vi "Teleop.vi"(10 "Match Info":T1={"Autonomous Elapsed Seconds"=0.0, "TeleOp Elapsed Seconds"=0.0, "Disabled Elapsed Seconds"=0.0, "Visited Autonomous"=FALSE, "Visited TeleOp"=FALSE, "Visited Disabled"=FALSE, "Autonomous Settings"={"Autonomous Style"=enum."Independent", "VI Refnum"=refnum}}, 11 "Call Context":T2) -> ()   [LabVIEW 2015]
doc: "This VI is called for each TeleOp packet received from the DS where the robot is not disabled. It is often used to read from the joysticks and update I/O or to update setpoints for timed control loops. It should complete and return within 20 milliseconds or it may miss DS packets."
uses:
  <vilib>/Rock Robotics/WPI/DriverStation/WPI_DriverStationDerivedRobotMode.ctl
  <vilib>/Rock Robotics/WPI/DriverStation/WPI_DriverStationMatch Info.ctl
  <vilib>/Rock Robotics/WPI/Utilities/WPI_GetSetVariantRefNum.vi
  Robot Global Data.vi
  <vilib>/Rock Robotics/Network Tables/NT Write Boolean Array.vi
  <vilib>/Rock Robotics/Network Tables/NT Write Numeric Array.vi
  <vilib>/Rock Robotics/Network Tables/NT Write Boolean.vi
  <vilib>/Rock Robotics/WPI/RobotDrive/WPI_RobotDriveArcadeDrive_Standard(NoSaturation).vi
  <vilib>/Rock Robotics/Network Tables/NT Read Boolean.vi
  <vilib>/Rock Robotics/Network Tables/NT Read Number.vi
panel:
  in  "command limit":dbl=0.25
  out "Sample Slider 0":dbl(slide) scale=0.0..5.0
  out "Sample Boolean 1":bool
  out "Sample Boolean 0":bool
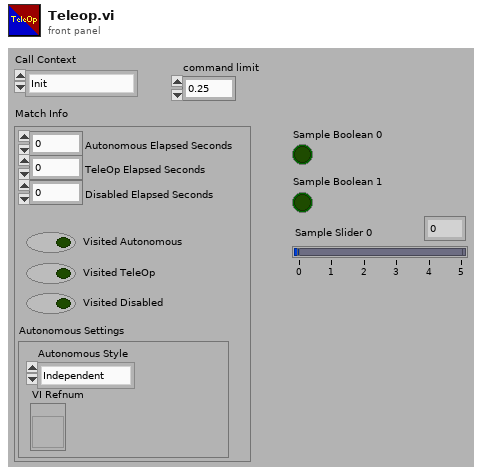
[diagram p1: front panel]
types:
  T1 = typedef "WPI_DriverStationMatch Info.ctl" = cluster{"Autonomous Elapsed Seconds":dbl, "TeleOp Elapsed Seconds":dbl, "Disabled Elapsed Seconds":dbl, "Visited Autonomous":bool, "Visited TeleOp":bool, "Visited Disabled":bool, "Autonomous Settings":cluster{"Autonomous Style":enum16{"Iterative", "Independent"}, "VI Refnum":refnum<vi>}}
  T2 = typedef "WPI_DriverStationDerivedRobotMode.ctl" = enum16{"Init", "Execute", "Stop"}
  T3 = typedef "WPI_JoystickDevRef.ctl" = cluster{"Device":T4}
  T4 = typedef "WPI_JoystickDeviceEnum.ctl" = enum16{"USB 0", "USB 1", "USB 2", "USB 3", "USB 4", "USB 5"}
  T5 = typedef "WPI_RobotDriveDevRef.ctl" = cluster{"DevStatus":errorcluster, "Motors[]":T6[], "Square Inputs":bool, "Max Output":dbl}
  T6 = typedef "WPI_MotorControlDeviceRef.ctl" = cluster{"DeviceStatus":errorcluster, "Type":T7, "PWM":cluster{"PWM Channel":T8, "DeadBand":T9}, "CAN":cluster{"Device Number":u8, "Control Mode":T10, "Semaphore":T11, "Max Vout":dbl, "TalonSRX Control Mode":T12}, "Invert":bool}
  T7 = typedef "WPI_MotorControlType.ctl" = enum16{"PWM", "CAN", "CANTalonSRX"}
  T8 = typedef "FPGA_DIOPWMChannel.ctl" = enum8{"PWM 0", "PWM 1", "PWM 2", "PWM 3", "PWM 4", "PWM 5", "PWM 6", "PWM 7", "PWM 8", "PWM 9", "PWM MXP 0", "PWM MXP 1", "PWM MXP 2", "PWM MXP 3", "PWM MXP 4", "PWM MXP 5", "PWM MXP 6", "PWM MXP 7", "PWM MXP 8", "PWM MXP 9", "Invalid"}
  T9 = typedef "WPI_PWMDeadband.ctl" = cluster{"Name":string, "maxPositivePwm":i32, "minPositivePwm":i32, "centerPwm":i32, "maxNegativePwm":i32, "minNegativePwm":i32, "angularRange":u16}
  T10 = typedef "WPI_CANJaguar_ControlMode.ctl" = enum8{"Percent VBus", "Current", "Speed", "Position", "Voltage"}
  T11 = typedef "Semaphore RefNum" = refnum<k1>
  T12 = typedef "WPI_CANTalonSRX_APIControlMode.ctl" = enum8{"Percent VBus", "Speed", "Position", "Slave", "Unchanged / Invalid", "Voltage Compensation", "Current", "Motion Profile"}
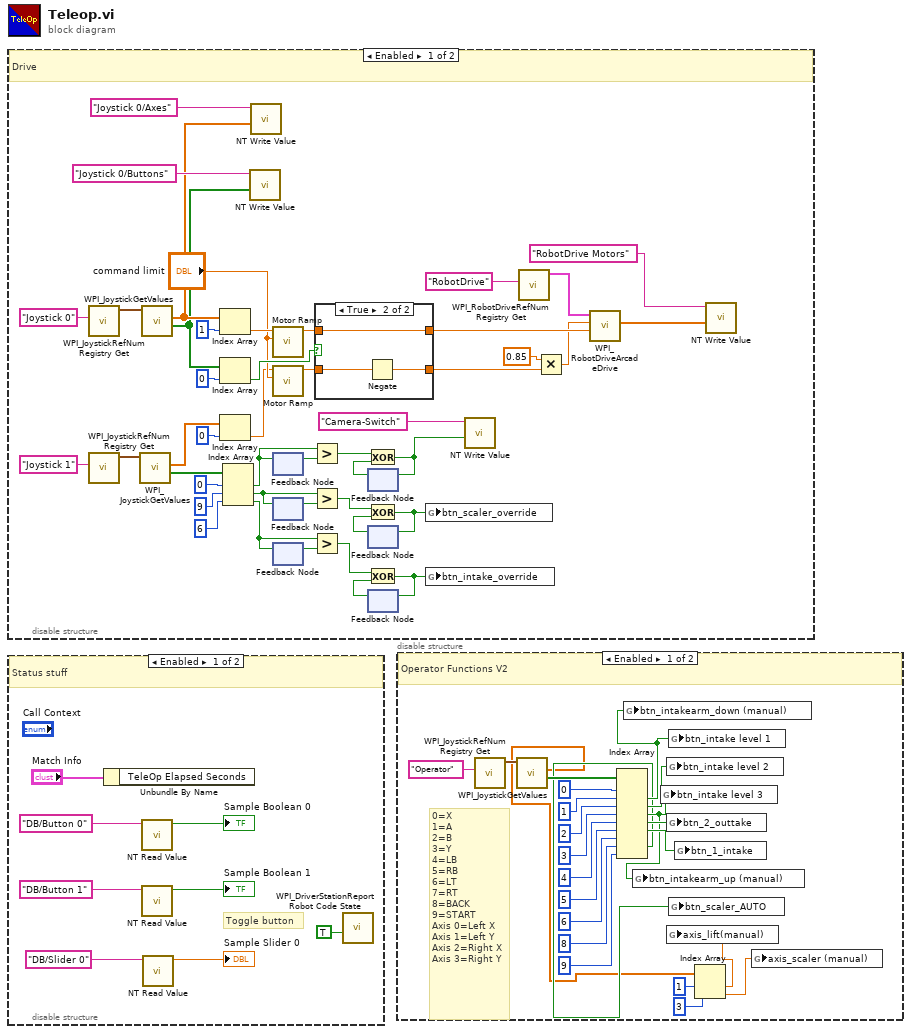
[diagram p0: block diagram]
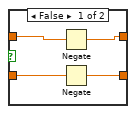
[diagram p3: hidden frame]
diagram:
  n1 = disable-structure shown="Enabled" {
    frame Enabled {
      # "Drive"
      n2 = call <vilib>:"WPI_JoystickRefNum Registry Get.vi"("refnum name"="Joystick 0") -> ("JoystickDevRef"=w44:T3)  [unwired: 1 in, 9 out]
      n3 = call <vilib>:"WPI_JoystickRefNum Registry Get.vi"("refnum name"="Joystick 1") -> ("JoystickDevRef"=w35:T3)  [unwired: 1 in, 9 out]
      n4 = call <vilib>:"WPI_JoystickGetValues.vi"("JoystickDevRef"=w35) -> ("Buttons"=w26:bool[], "Axes"=w34:dbl[])  [unwired: 6 in, 3 out]
      n5 = call <vilib>:"WPI_JoystickGetValues.vi"("JoystickDevRef"=w44) -> ("Buttons"=w40:bool[], "Axes"=w41:dbl[])  [unwired: 6 in, 3 out]
      n6 = Index Array(array=w41, index=1) -> (element=w20:dbl)
      n7 = Index Array(array=w40, index=0) -> (element=w23:bool)
      n8 = Index Array(array=w34, index=0) -> (element=w17:dbl)
      n9 = Index Array(array=w26, index #1=0 ("index"), index #2=9 ("index"), index #3=6 ("index")) -> (element #1=w27:bool, element #2=w8:bool, element #3=w1:bool)
      n10 = call-poly <vilib>:"NT Write Value.vi"("Boolean Array"=w40, "Name"="Joystick 0/Buttons") -> ()  [unwired: 9 in, 1 out]
      n11 = call-poly <vilib>:"NT Write Value.vi"("Numeric Array"=w41, "Name"="Joystick 0/Axes") -> ()  [unwired: 9 in, 1 out]
      n12 = call "Motor Ramp.vi"("Command limit"="command limit", "Joystick in"=w20) -> ("Joystick out"=w21:dbl)  [unwired: 9 in]
      n13 = call "Motor Ramp.vi"("Command limit"="command limit", "Joystick in"=w17) -> ("Joystick out"=w18:dbl)  [unwired: 9 in]
      n14 = feedback #1() -> (w28:bool)  [unwired: 1 in]
      n15 = feedback-in #1(w27) -> ()
      n16 = feedback #2() -> (w12:bool)  [unwired: 1 in]
      n17 = feedback-in #2(w8) -> ()
      n18 = feedback #3() -> (w2:bool)  [unwired: 1 in]
      n19 = feedback-in #3(w1) -> ()
      n20 = Greater?(x=w27, y=w28) -> (0:w29:bool)
      n21 = Greater?(x=w8, y=w12) -> (0:w7:bool)
      n22 = Greater?(x=w1, y=w2) -> (0:w4:bool)
      n23 = case shown="True" w23 {
        tunnel: w21 -> [w49 w53]
        tunnel: w18 -> [w50 w52]
        tunnel: [w48 w51] -> w15
        tunnel: [w47 w53] -> w16
        frame False {
          n24 = Negate(x=w49) -> (-x=w47:dbl)
          n25 = Negate(x=w50) -> (-x=w48:dbl)
        }
        frame True {
          n26 = Negate(x=w52) -> (-x=w51:dbl)
        }
      }
      n27 = feedback #4() -> (w30:bool)  [unwired: 1 in]
      n28 = Exclusive Or(1:w30, 2:w29) -> (0:w31:bool)
      n29 = feedback-in #4(w31) -> ()
      n30 = feedback #5() -> (w11:bool)  [unwired: 1 in]
      n31 = Exclusive Or(1:w11, 2:w7) -> (0:w6:bool)
      n32 = feedback-in #5(w6) -> ()
      n33 = feedback #6() -> (w3:bool)  [unwired: 1 in]
      n34 = Exclusive Or(1:w3, 2:w4) -> (0:w5:bool)
      n35 = feedback-in #6(w5) -> ()
      n36 = global write "Robot Global Data.vi" "btn_scaler_override"(w6) -> ()
      n37 = global write "Robot Global Data.vi" "btn_intake_override"(w5) -> ()
      n38 = call-poly <vilib>:"NT Write Value.vi"("Boolean"=w31, "Name"="Camera-Switch") -> ()  [unwired: 9 in, 1 out]
      n39 = call <vilib>:"WPI_RobotDriveRefNum Registry Get.vi"("refnum name"="RobotDrive") -> ("RobotDriveDevRef"=w46:T5)  [unwired: 1 in, 9 out]
      n40 = Multiply(x=0.85, y=w15) -> (x*y=w14:dbl)
      n41 = call-poly <vilib>:"WPI_RobotDriveArcadeDrive.vi"("Y axis value"=w16, "X axis value"=w14, "RobotDriveDevRef"=w46) -> ("Motor Values"=w39:dbl[])  [unwired: 6 in, 2 out]
      n42 = call-poly <vilib>:"NT Write Value.vi"("Numeric Array"=w39, "Name"="RobotDrive Motors") -> ()  [unwired: 9 in, 1 out]
    }
    frame Disabled {
    }
  }
  n43 = disable-structure shown="Enabled" {
    frame Enabled {
      # "Toggle button"
      # "Status stuff"
      n44 = Unbundle By Name("Match Info") -> ()  [unwired: 1 out]
      n45 = call-poly <vilib>:"NT Read Value.vi"("Name"="DB/Button 0" ("refnum name")) -> ("Boolean"=→"Sample Boolean 0":bool)  [unwired: 9 in, 1 out]
      n46 = call-poly <vilib>:"NT Read Value.vi"("Name"="DB/Button 1" ("refnum name")) -> ("Boolean"=→"Sample Boolean 1":bool)  [unwired: 9 in, 1 out]
      n47 = call-poly <vilib>:"NT Read Value.vi"("Name"="DB/Slider 0" ("refnum name")) -> ("Numeric"=→"Sample Slider 0":dbl)  [unwired: 9 in, 1 out]
      n48 = call <vilib>:"WPI_DriverStationReport Robot Code State.vi"("TeleOp"=TRUE ("Autonomous")) -> ()  [unwired: 10 in, 1 out]
    }
    frame Disabled {
    }
  }
  n49 = disable-structure shown="Enabled" {
    frame Enabled {
      # "0=X\n1=A\n2=B\n3=Y\n4=LB\n5=RB\n6=LT\n7=RT\n8=BACK\n9=START\nAxis 0=Left X\nAxis 1=Left Y\nAxis 2=Right X\nAxis 3=Right Y"
      # "Operator Functions V2"
      n50 = call <vilib>:"WPI_JoystickRefNum Registry Get.vi"("refnum name"="Operator") -> ("JoystickDevRef"=w83:T3)  [unwired: 1 in, 9 out]
      n51 = call <vilib>:"WPI_JoystickGetValues.vi"("JoystickDevRef"=w83) -> ("Buttons"=w81:bool[], "Axes"=w66:dbl[])  [unwired: 6 in, 3 out]
      n52 = Index Array(array=w81, index #1=0 ("index"), index #2=1 ("index"), index #3=2 ("index"), index #4=3 ("index"), index #5=4 ("index"), index #6=5 ("index"), index #7=6 ("index"), index #8=8 ("index"), index #9=9 ("index")) -> (element #2=w69:bool, element #3=w78:bool, element #4=w68:bool, element #5=w75:bool, element #6=w73:bool, element #8=w67:bool)  [unwired: 3 out]
      n53 = global write "Robot Global Data.vi" "btn_intakearm_down (manual)"(w69) -> ()
      n54 = global write "Robot Global Data.vi" "btn_intakearm_up (manual)"(w68) -> ()
      n55 = global write "Robot Global Data.vi" "btn_intake level 3"(w68) -> ()
      n56 = global write "Robot Global Data.vi" "btn_intake level 2"(w78) -> ()
      n57 = global write "Robot Global Data.vi" "btn_2_outtake"(w75) -> ()
      n58 = global write "Robot Global Data.vi" "btn_intake level 1"(w69) -> ()
      n59 = global write "Robot Global Data.vi" "btn_scaler_AUTO"(w67) -> ()
      n60 = global write "Robot Global Data.vi" "btn_1_intake"(w73) -> ()
      n61 = Index Array(array=w66, index #1=1 ("index"), index #2=3 ("index")) -> (element #1=w65:dbl, element #2=w64:dbl)
      n62 = global write "Robot Global Data.vi" "axis_lift(manual)"(w65) -> ()
      n63 = global write "Robot Global Data.vi" "axis_scaler (manual)"(w64) -> ()
    }
    frame Disabled {
    }
  }
